vi "SaveDATA.vi"(8 "error in (no error)":errorcluster, 10 "Numeric":dbl, 11 "Loggin in":refnum<class "Loggin.lvclass">) -> (0 "error out":errorcluster, 3 "Loggin out":refnum<class "Loggin.lvclass">)   [LabVIEW 2020, in "TDMS.lvlib" / "TDMS.lvclass"]
uses:
  TDMS.lvclass
  Loggin/Loggin/Loggin.lvclass
  Loggin/Loggin/Loggin.lvclass/Loggin.ctl
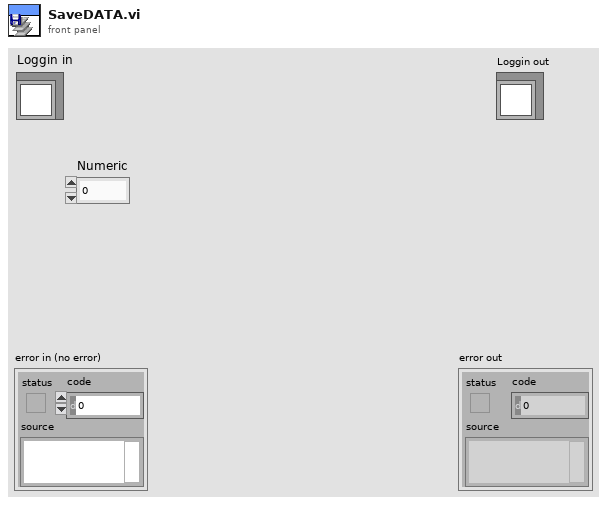
[diagram p1: front panel]
types:
  T1 = enum16{"open", "open or create", "create or replace", "create", "open (read-only)"}
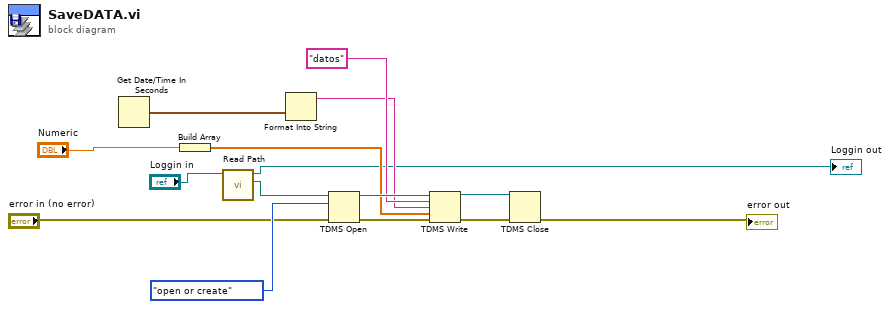
[diagram p0: block diagram]
diagram:
  n1 = Get Date/Time In Seconds() -> (seconds since 1Jan1904=w3:timestamp)
  n2 = Build Array("Numeric") -> (w10:dbl[])
  n3 = call "Read Path.vi"("Loggin in"="Loggin in") -> ("Path"=w5:path, "Loggin out"=→"Loggin out":refnum<class "Loggin.lvclass">)  [unwired: 8 in, 1 out]
  n4 = Format Into String(w3) -> (resulting string=w4:string)  [unwired: 3 in, 1 out]
  n5 = TDMS Open(8:"error in (no error)", 10:T1."open or create" ("operation (0:open)"), 11:w5) -> (0:w14:errorcluster, 3:w15:refnum<k34>)  [unwired: 4 in]
  n6 = TDMS Write(0:w15, 5:"datos" ("group name in (Untitled)"), 7:w4, 9:w10, 11:w14) -> (4:w13:refnum<k34>, 15:w12:errorcluster)  [unwired: 1 in, 2 out]
  n7 = TDMS Close(8:w12, 11:w13) -> (0:→"error out":errorcluster)  [unwired: 1 out]
